vi "Send Channel List Update.vi"(8 "error in (no error)":errorcluster, 11 "CIFChannelMng in":refnum<class "CIFChannelMng.lvclass">) -> (0 "error out":errorcluster, 3 "CIFChannelMng out":refnum<class "CIFChannelMng.lvclass">)   [LabVIEW 2021, in "CIFChannelMng.lvclass"]
uses:
  CIFChannelMng.lvclass
  CIFChannelMng.lvclass/CIFChannelMng.ctl
  typedef/TX CIPC Data.ctl
  typedef/TX Commands.ctl
  463ebf4c-8748-40f9-8ad3-9e61c16a01a6.vi
  <vilib>/CIF Foundation/CIF CIPC/SubVIs/Check Error.vi
  <vilib>/CIF Foundation/CIF CIPC/SubVIs/Get Element Write Position.vi
  <vilib>/CIF Foundation/CIF CIPC/SubVIs/Notify Of New Write.vi
  <vilib>/CIF Foundation/CIF CIPC/SubVIs/Get dll Path.vi
  <vilib>/CIF Foundation/CIF CIPC/SubVIs/Get Element Info Variant.vi
  <vilib>/Utility/error.llb/Trim Whitespace.vi
  <vilib>/Utility/error.llb/Error Cluster From Error Code.vi
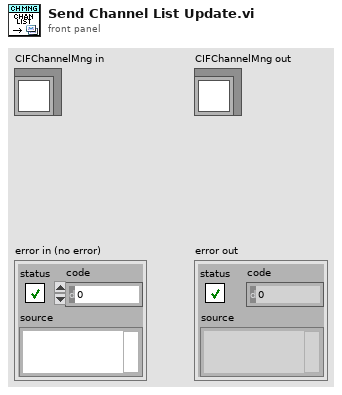
[diagram p1: front panel]
types:
  T1 = typedef "CIFChannelMng.lvclass/TX CIPC Data.ctl" = cluster{"TX Commands":T2}
  T2 = typedef "CIFChannelMng.lvclass/TX Commands.ctl" = enum8{"Channel List", "New FIFO Pub"}
  T3 = typedef "CIFChannelMng.lvclass/Channel List for OOB.ctl" = cluster{"Name":string, "Direction":T4, "Type":string, "Connected?":bool, "Connected Name":string, "Custom Config Data":u8[], "Forced?":bool, "Pattern":T5}
  T4 = typedef "CIFChannels.lvclass/Direction.ctl" = enum16{"Publisher", "Subscriber"}
  T5 = typedef "ChannelCommon.lvlib/Channel Pattern.ctl" = enum16{"Unknown", "Tag", "FIFO", "MultiFIFO"}
  T6 = typedef "CIFChannelMng.lvclass/TX DVR Data.ctl" = cluster{"Channel List":T3[], "Publisher Instance":T7}
  T7 = typedef "CIFChannelMng.lvclass/FIFO Publisher Return.ctl" = cluster{"FIFO Pub Name":string, "error":errorcluster, "Added":bool}
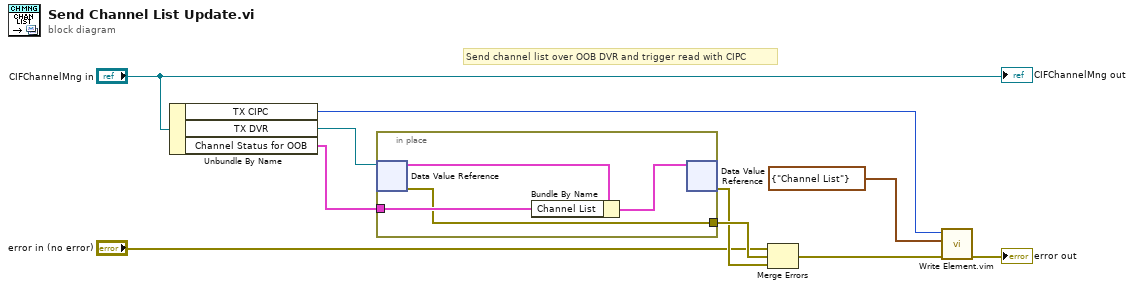
[diagram p0: block diagram]
diagram:
  # "Send channel list over OOB DVR and trigger read with CIPC"
  n1 = Unbundle By Name("CIFChannelMng in") -> ("TX CIPC"=w10:u64, "TX DVR"=w2:refnum<data-value>, "Channel Status for OOB"=w1:T3[])
  n2 = in-place {
    in-place-border: w1 -> [w12]
    in-place-border: [w11] -> w7
    n3 = in-place-dvr #1(w2) -> (w14:T6, w11:errorcluster)
    n4 = Bundle By Name(cluster=w14, "Channel List"=w12) -> (w13:T6)
    n5 = in-place-dvr #1(w13) -> (w6:errorcluster)  [unwired: 1 out]
  }
  n6 = Merge Errors("error in (no error)", w7, w6) -> (w3:errorcluster)
  n7 = call "Write Element.vim"("error in (no error)"=w3, "Data in"=T1 {"TX Commands"=enum."Channel List"}, "CIPC Reference in"=w10) -> ("error out"=→"error out":errorcluster)  [unwired: 5 in, 3 out]
  "CIFChannelMng out" <- "CIFChannelMng in"
